vi "Zip.vi"(8 "error in":errorcluster, 11 "Archivist in":refnum<class "Archivist.lvclass">) -> (0 "error out":errorcluster, 2 "archive name out":path, 3 "Archivist out":refnum<class "Archivist.lvclass">)   [LabVIEW 2019, in "Archivist.lvclass"]
uses:
  Archivist.lvclass
  <userlib>/_OpenG.lib/lvzip/lvzip.llb/subVI/ZLIB Compress Directory (Path)__ogtk.vi
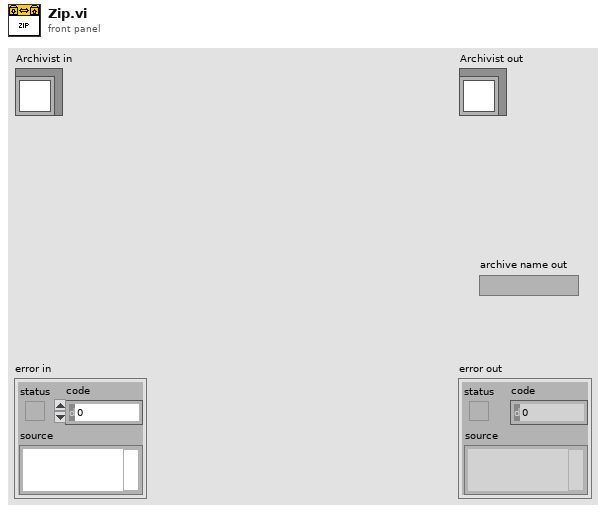
[diagram p1: front panel]
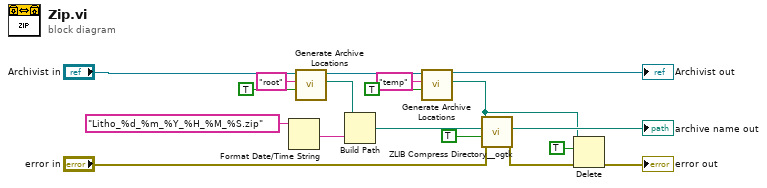
[diagram p0: block diagram]
diagram:
  n1 = Format Date/Time String(time format string (%c)="Litho_%d_%m_%Y_%H_%M_%S.zip") -> (date/time string=w2:string)  [unwired: 2 in]
  n2 = call "Generate Archive Locations.vi"("Archive?"=TRUE, "Key"="root", "Archivist In"="Archivist in") -> ("Path Out"=w3:path, "Archivist Out"=w4:refnum<class "Archivist.lvclass">)  [unwired: 7 in]
  n3 = Build Path(base path=w3, name or relative path=w2) -> (appended path=w1:path)
  n4 = call "Generate Archive Locations.vi"("Archive?"=TRUE, "Key"="temp", "Archivist In"=w4) -> ("Path Out"=w12:path, "Archivist Out"=→"Archivist out":refnum<class "Archivist.lvclass">)  [unwired: 7 in]
  n5 = call-poly <userlib>:"ZLIB Compress Directory__ogtk.vi"("error in (no error)"="error in", "include subdirectories (F)"=TRUE, "archive name (root directory with .zip ending)"=w1, "root directory (file dialog)"=w12) -> ("error out"=w8:errorcluster, "archive name out"=→"archive name out":path)  [unwired: 5 in, 1 out]
  n6 = Delete(path (use dialog)=w12, entire hierarchy (F)=TRUE, error in=w8) -> (error out=→"error out":errorcluster)  [unwired: 2 in, 2 out]
